vi "Read Strategies.vi"(11 "Banana in":refnum<class "Banana.lvclass">) -> (1 "Strategies":T1, 3 "Banana out":refnum<class "Banana.lvclass">)   [LabVIEW 2021, in "Bananas.lvlib" / "Banana.lvclass"]
uses:
  Banana.lvclass
  Assertion Strategies -- cluster.ctl
  AssertTrue/AssertTrue.lvclass
  Banana.lvclass/Banana.ctl
  Bananas.lvlib
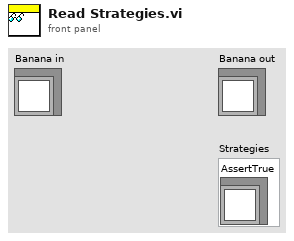
[diagram p1: front panel]
types:
  T1 = typedef "Bananas.lvlib/Assertion Strategies -- cluster.ctl" = cluster{"AssertTrue":refnum<class "AssertTrue.lvclass">}
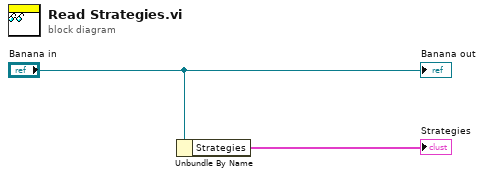
[diagram p0: block diagram]
diagram:
  n1 = Unbundle By Name("Banana in") -> ("Strategies"=→"Strategies":T1)
  "Banana out" <- "Banana in"
